vi "ERD Read Test Generic (Uint).vi"(0 "GEA2 Reference In":refnum<k24>, 1 "Expected Value (Dec)":u32, 5 "Standalone?":bool, 7 "ERD Number":u16=61699 format="%.0x", 9 "Data Type":T1(ring)=enum."boolean", 11 "Error In":errorcluster) -> (4 "GEA2 Reference Out":refnum<k24>, 6 "Pass/Fail?":bool, 15 "Error Out":errorcluster)   [LabVIEW 2016, in "TL27.lvlib"]
uses:
  Projects/TL27.lvlib
  C:/Automation/DLLs/PC Dot Net/GeaCommunication.dll
  Common/LabVIEW GEA2 Toolkit/LabVIEW_GEA2_Toolkit.lvlibp/type defs/Source_Destination.ctl
  Common/LabVIEW GEA2 Toolkit/LabVIEW_GEA2_Toolkit.lvlibp/type defs/ERD Read Data In.ctl
  Common/LabVIEW GEA2 Toolkit/LabVIEW_GEA2_Toolkit.lvlibp/type defs/Data Type.ctl
  Common/LabVIEW GEA2 Toolkit/LabVIEW_GEA2_Toolkit.lvlibp
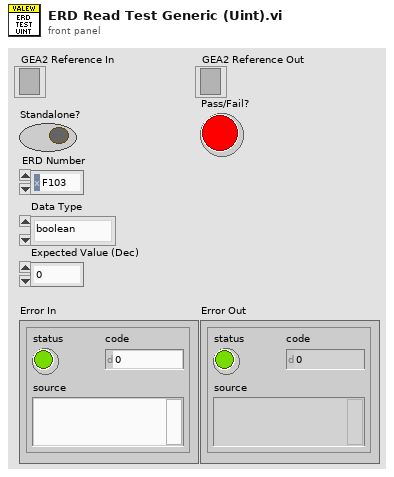
[diagram p1: front panel]
types:
  T1 = enum16{"string", "boolean", "uint8_t", "uint16_t", "uint32_t"}
  T2 = typedef "LabVIEW_GEA2_Toolkit.lvlibp/ERD Read Data In.ctl" = cluster{"ERD Number":u16, "Data Type":T3}
  T3 = typedef "LabVIEW_GEA2_Toolkit.lvlibp/Data Type.ctl" = enum16{"string", "boolean", "uint8_t", "uint16_t", "uint32_t", "uint64_t", "int8_t", "int16_t", "int32_t", "int64_t"}
  T4 = typedef "LabVIEW_GEA2_Toolkit.lvlibp/Source_Destination.ctl" = cluster{"Source":u8, "Destination":u8}
  T5 = typedef "LabVIEW_GEA2_Toolkit.lvlibp/ERD Read Data Out.ctl" = cluster{"ERD Number":u16, "Data":string}
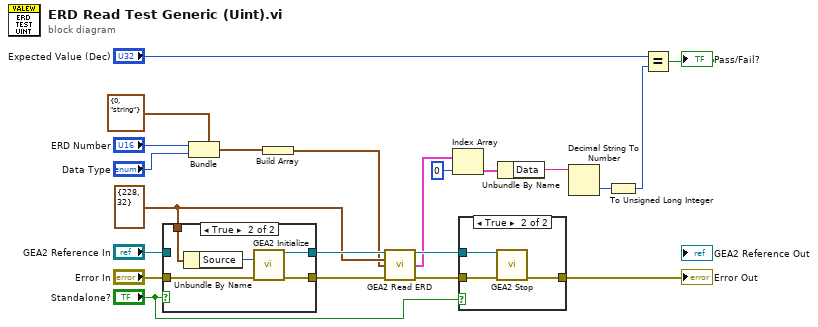
[diagram p0: block diagram]
diagram:
  w14 = T4 {"Source"=228, "Destination"=32} ("GEA Inputs")
  n1 = case shown="True" "Standalone?" {
    tunnel: "Error In" -> [w23 w29]
    tunnel: [w23 w28] -> w18
    tunnel: "GEA2 Reference In" -> [w24 _]
    tunnel: [w24 w27] -> w16
    tunnel: w14 -> [_ w25]
    frame False {
    }
    frame True {
      n2 = Unbundle By Name(w25) -> ("Source"=w26:u8)
      n3 = call "GEA2 Initialize.vi"("Source Address"=w26, "error in"=w29) -> ("GEA2 Reference Out"=w27:refnum<k24>, "error out"=w28:errorcluster)  [unwired: 11 in, 1 out]
    }
  }
  n4 = Bundle(cluster=T2 {"ERD Number"=0, "Data Type"=enum."string"} ("ERD Read Data In"), "ERD Number"="ERD Number", "Data Type"="Data Type") -> (w3:T2)
  n5 = Build Array(w3) -> (w2:T2[])
  n6 = call "GEA2 Read ERD.vi"("GEA2 Reference In"=w16, "GEA Inputs"=w14, "Read ERD List"=w2, "Error In"=w18) -> ("GEA2 Reference Out"=w15:refnum<k24>, "ERD Data Out"=w13:T5[], "Error Out"=w17:errorcluster)  [unwired: 8 in, 1 out]
  n7 = Index Array(array=w13, index=0) -> (element=w11:T5)
  n8 = case shown="True" "Standalone?" {
    tunnel: [w30 w33] -> w20
    tunnel: w17 -> [w30 w32]
    tunnel: w15 -> [_ w31]
    frame False {
    }
    frame True {
      n9 = call "GEA2 Stop.vi"("GEA2 Reference In"=w31, "Error In"=w32) -> ("Error Out"=w33:errorcluster)  [unwired: 13 in]
    }
  }
  "Error Out" <- w20
  n10 = Unbundle By Name(w11) -> ("Data"=w10:string)
  n11 = Decimal String To Number(string=w10) -> (number=w8:i32)  [unwired: 2 in, 1 out]
  n12 = To Unsigned Long Integer(number=w8) -> (unsigned 32bit integer=w7:u32)
  n13 = Equal?(x="Expected Value (Dec)", y=w7) -> (x = y?=→"Pass/Fail?":bool)
